vi "Different Star Pattern.vi"() -> ()   [LabVIEW 2015]
panel:
  out "part 1":string
  out "concatenated string":string
  in  "stop":bool
  out "reversed":string
  out "Part 2":string
  # "Different Star Pattern"
  # "Pardeep Kumar"
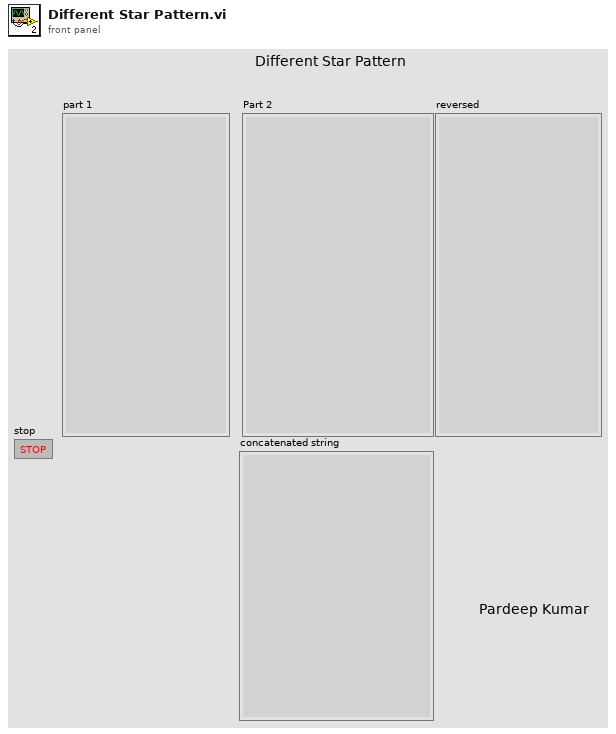
[diagram p1: front panel]
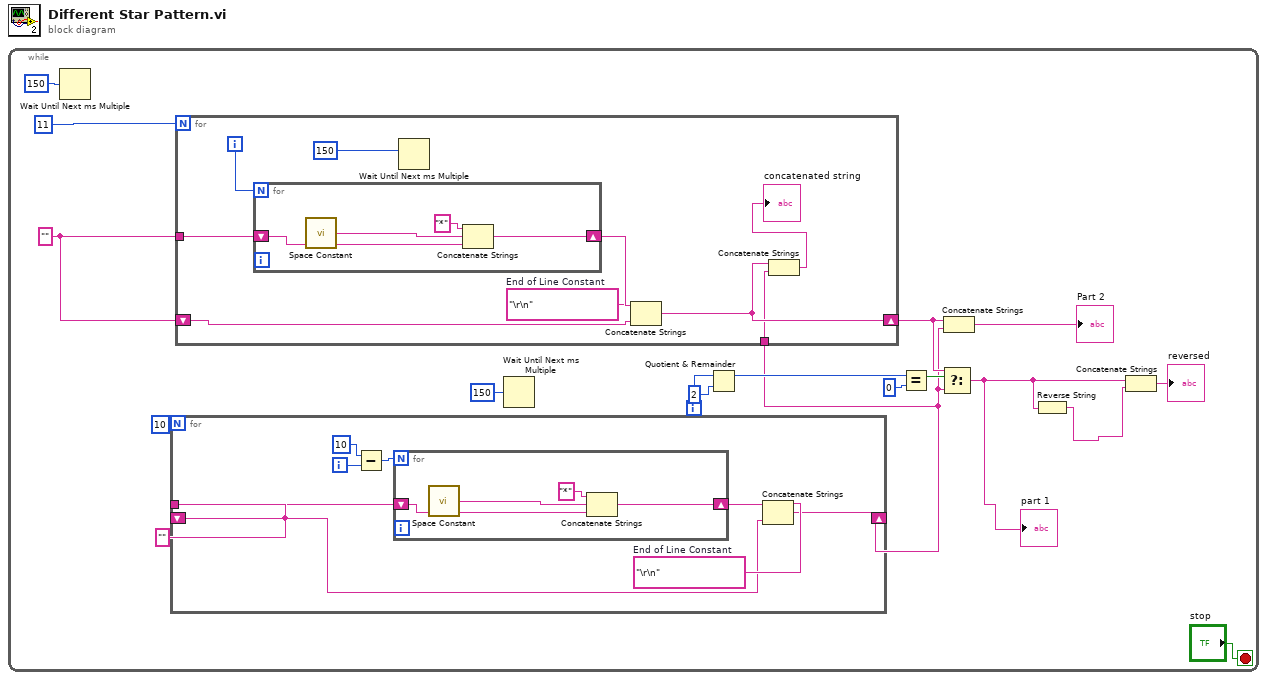
[diagram p0: block diagram]
diagram:
  n1 = while {
    i -> [w9]
    stop <- "stop" stop-if-true
    w15 = ""
    w17 = ""
    n2 = Wait Until Next ms Multiple(millisecond multiple=u32 150) -> ()  [unwired: 1 out]
    n3 = for {
      N: 10 -> [_]
      shift-right: [w19] -> w1
      shift-left: w15 -> [w24]
      tunnel: w15 -> [w23]
      i -> [w20]
      w25 = "\r\n"  # End of Line Constant
      n4 = Subtract(x=10 ("y"), y=w20) -> (x-y=w22:i32)
      n5 = for {
        N: w22 -> [_]
        shift-right: [w28] -> w26
        shift-left: w23 -> [w27]
        n6 = call <vilib>:"Space Constant.vi"() -> ("String"=w29:string)
        n7 = Concatenate Strings "Concatenate Strings"("*" ("string"), w29, w27) -> (w28:string)
      }
      n8 = Concatenate Strings "Concatenate Strings"(w26, w25, w24) -> (w19:string)
    }
    n9 = for {
      N: 11 -> [_]
      shift-right: [w33] -> w13
      shift-left: w17 -> [w37]
      tunnel: w17 -> [w36]
      tunnel: w1 -> [w31]
      i -> [w35]
      w38 = "\r\n"  # End of Line Constant
      n10 = for {
        N: w35 -> [_]
        shift-right: [w41] -> w39
        shift-left: w36 -> [w40]
        n11 = call <vilib>:"Space Constant.vi"() -> ("String"=w42:string)
        n12 = Concatenate Strings "Concatenate Strings"("*" ("string"), w42, w40) -> (w41:string)
      }
      n13 = Wait Until Next ms Multiple(millisecond multiple=u32 150) -> ()  [unwired: 1 out]
      n14 = Concatenate Strings "Concatenate Strings"(w39, w38, w37) -> (w33:string)
      n15 = Concatenate Strings "Concatenate Strings"(w33, w31) -> (→"concatenated string":string)
    }
    n16 = Wait Until Next ms Multiple(millisecond multiple=u32 150) -> ()  [unwired: 1 out]
    n17 = Quotient & Remainder(x=w9, y=2) -> (x-y*floor(x/y)=w7:i32)  [unwired: 1 out]
    n18 = Equal?(x=w7, y=0) -> (x = y?=w5:bool)
    n19 = Select(t=w13, s=w5, f=w1) -> (s? t:f=w11:string)
    "part 1" <- w11
    n20 = Concatenate Strings "Concatenate Strings"(w13, w1) -> (→"Part 2":string)
    n21 = Reverse String(1:w11) -> (0:w2:string)
    n22 = Concatenate Strings(w11, w2) -> (→"reversed":string)
  }
